vi "AE.vi"() -> ()   [LabVIEW 2012]
uses:
  <vilib>/DAQmx/read.llb/DAQmx Read (Analog 1D Wfm NChan NSamp).vi
  <vilib>/DAQmx/create/channels.llb/DAQmx Create Channel (AI-Voltage-Basic).vi
  <vilib>/DAQmx/configure/timing.llb/DAQmx Timing (Sample Clock).vi
  <vilib>/DAQmx/miscellaneous.llb/DAQmx Fill In Error Info.vi
panel:
  in  "Physical Channel":tag="Dev1/ai0"
  in  "Gain":u16(ring)=1 items=["20 dB", "40 dB", "60 dB"]
  out "Events":i32
  in  "Sample Window (us)":i32=200 min=0 max=1000
  in  "stop":bool
  in  "Test Name":string="test"
  in  "Storage Directory":path=path "C:/Users/User/Desktop/Users_2013-2014/Michael Rossol"
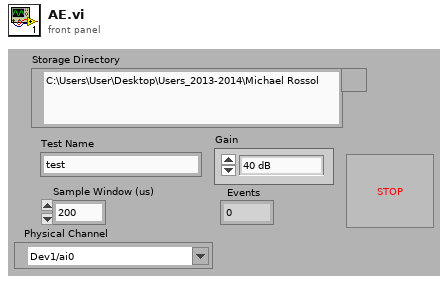
[diagram p1: front panel]
types:
  T1 = enum16{"open", "open or create", "create or replace", "create", "open (read only)"}
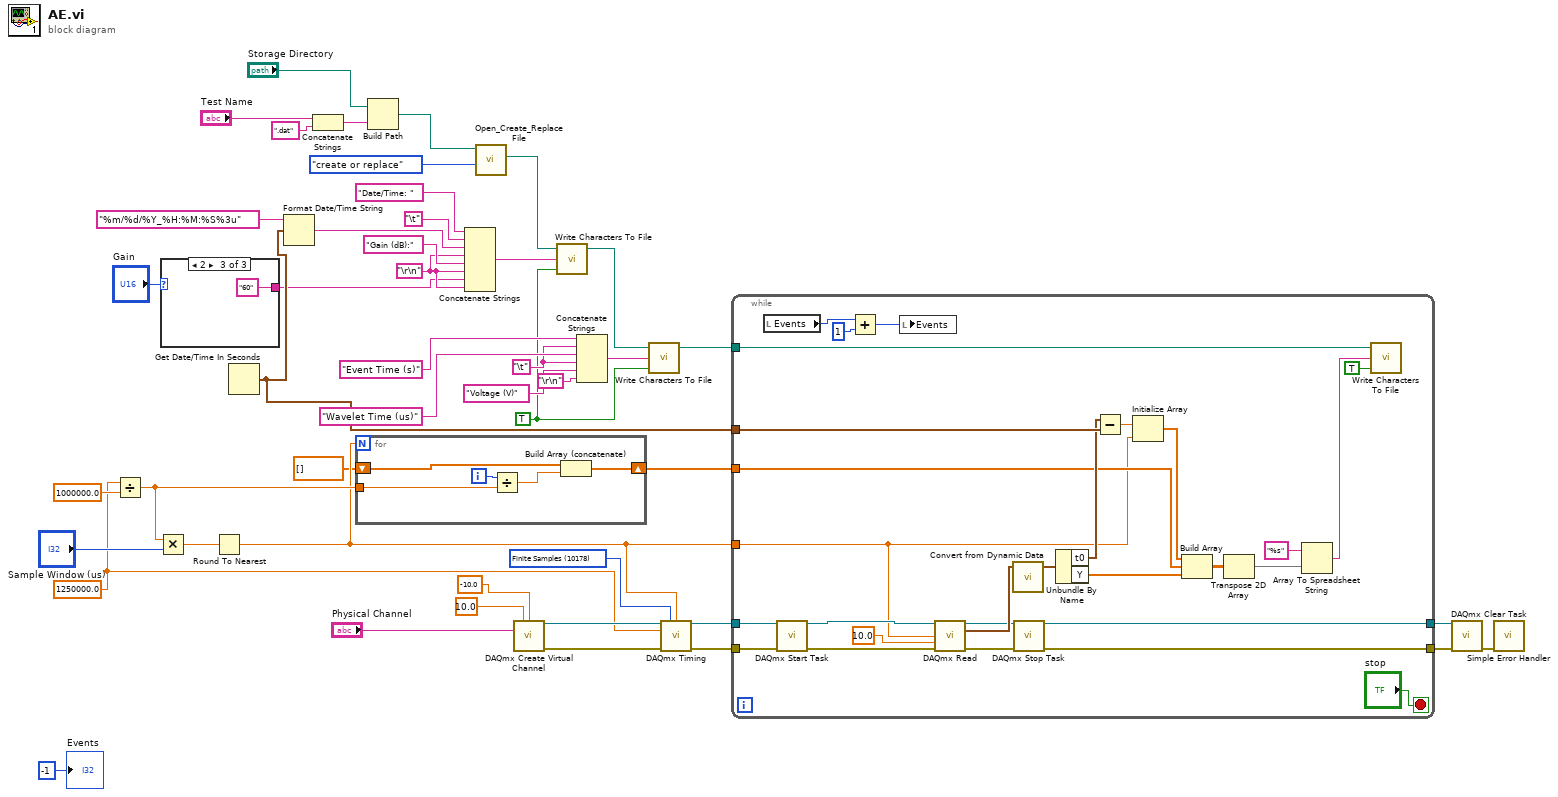
[diagram p0: block diagram]
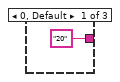
[diagram p2: hidden frame]
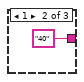
[diagram p3: hidden frame]
diagram:
  w11 = 10178 items=["Finite Samples"=10178, "Continuous Samples"=10123] ("sample mode")
  w27 = "\t"
  w10 = 1250000.0 ("x")
  w19 = "\r\n"
  w24 = TRUE ("append to file? (new file:F)")
  n1 = Divide(x=w10, y=1000000.0) -> (x/y=w30:dbl)
  n2 = Multiply(x=w30, y="Sample Window (us)") -> (x*y=w4:dbl)
  n3 = case shown="2" "Gain" {
    tunnel: ["20" ("string") "40" ("string") "60" ("string")] -> w17
    frame 0, Default {
    }
    frame 1 {
    }
    frame 2 {
    }
  }
  n4 = Round To Nearest(number=w4) -> (nearest integer value=w3:dbl)
  n5 = Get Date/Time In Seconds() -> (seconds since 1Jan1904=w32:timestamp)
  n6 = Format Date/Time String(time format string (%c)="%m/%d/%Y_%H:%M:%S%3u", seconds (now)=w32) -> (date/time string=w36:string)  [unwired: 1 in]
  n7 = Concatenate Strings("Test Name", ".dat" ("string")) -> (w39:string)
  n8 = for {
    N: w3 -> [_]
    shift-right: [w53] -> w2
    shift-left: dbl[] [] -> [w54]
    tunnel: w30 -> [w50]
    i -> [w52]
    n9 = Divide(x=w52, y=w50) -> (x/y=w51:dbl)
    n10 = Build Array (concatenate)(w54, w51) -> (w53:dbl[])
  }
  n11 = Build Path(base path="Storage Directory", name or relative path=w39) -> (appended path=w37:path)
  n12 = Concatenate Strings("Date/Time: ", "\t", w36, w19, "Gain (dB):" ("string"), w19, w17, w19) -> (w46:string)
  n13 = call <vilib>:"Open_Create_Replace File.vi"("function (open:0)"=T1."create or replace", "file path"=w37) -> ("new file path"=w42:path)  [unwired: 6 in, 3 out]
  n14 = call-poly <vilib>:"DAQmx Create Virtual Channel.vi"("maximum value"=10.0, "minimum value"=-10.0, "physical channels"="Physical Channel") -> ("task out"=w13:refnum<k21>, "error out"=w12:errorcluster)  [unwired: 11 in]
  n15 = call <vilib>:"Write Characters To File.vi"("append to file? (new file:F)"=w24, "character string"=w46, "file path (dialog if empty)"=w42) -> ("new file path (Not A Path if cancelled)"=w22:path)  [unwired: 2 in]
  n16 = Concatenate Strings("Event Time (s)" ("string"), w27, "Wavelet Time (us)" ("string"), w27, "Voltage (V)" ("string"), "\r\n") -> (w23:string)
  n17 = call <vilib>:"Write Characters To File.vi"("append to file? (new file:F)"=w24, "character string"=w23, "file path (dialog if empty)"=w22) -> ("new file path (Not A Path if cancelled)"=w21:path)  [unwired: 2 in]
  n18 = call-poly <vilib>:"DAQmx Timing.vi"("task/channels in"=w13, "sample mode"=w11, "samples per channel"=w3, "rate"=w10, "error in"=w12) -> ("task out"=w9:refnum<k21>, "error out"=w8:errorcluster)  [unwired: 9 in]
  n19 = while {
    tunnel: w21 -> [w79]
    tunnel: w3 -> [w61]
    tunnel: w32 -> [w73]
    tunnel: w2 -> [w67]
    tunnel: w9 -> [w64]
    tunnel: w8 -> [w63]
    tunnel: [w57] -> w6
    tunnel: [w56] -> w5
    stop <- "stop" stop-if-true
    n20 = local read "Events"() -> (w77:i32)
    n21 = call <vilib>:"DAQmx Start Task.vi"("task/channels in"=w64, "error in"=w63) -> ("task out"=w66:refnum<k21>, "error out"=w65:errorcluster)  [unwired: 12 in]
    n22 = Add(x=w77, y=1) -> (x+y=w76:i32)
    n23 = local write "Events"(w76) -> ()
    n24 = call-poly <vilib>:"DAQmx Read.vi"("task/channels in"=w66, "number of samples per channel"=w61, "timeout"=10.0, "error in"=w65) -> ("task out"=w58:refnum<k21>, "data"=w62:waveform(dbl)[], "error out"=w59:errorcluster)  [unwired: 9 in]
    n25 = call "Convert from Dynamic Data"("Dynamic Data Type"=w62) -> ("Waveform"=w74:waveform(dbl))  [unwired: 3 in]
    n26 = call <vilib>:"DAQmx Stop Task.vi"("task/channels in"=w58, "error in"=w59) -> ("task out"=w56:refnum<k21>, "error out"=w57:errorcluster)  [unwired: 12 in]
    n27 = Unbundle By Name(w74) -> ("t0"=w72:timestamp, "Y"=w55:dbl[])
    n28 = Subtract(x=w72, y=w73) -> (x-y=w71:dbl)
    n29 = Initialize Array(w71, w61) -> (w70:dbl[])
    n30 = Build Array(w70, w67, w55) -> (w69:dbl[][])
    n31 = Transpose 2D Array(2D array=w69) -> (transposed array=w68:dbl[][])
    n32 = Array To Spreadsheet String(array=w68, 3:"%s" ("format string")) -> (spreadsheet string=w80:string)  [unwired: 1 in]
    n33 = call <vilib>:"Write Characters To File.vi"("append to file? (new file:F)"=TRUE, "character string"=w80, "file path (dialog if empty)"=w79) -> ()  [unwired: 2 in, 1 out]
  }
  n34 = call <vilib>:"DAQmx Clear Task.vi"("task in"=w5, "error in"=w6) -> ("error out"=w7:errorcluster)  [unwired: 13 in]
  n35 = call <vilib>:"Simple Error Handler.vi"("error in (no error)"=w7) -> ()  [unwired: 4 in, 5 out]
  "Events" <- -1
